vi "ArcadeJoystick.vi"(6 "Max Output":dbl=1.0, 7 "Square Inputs":bool=TRUE, 9 "Y axis value":dbl, 10 "X axis value":dbl) -> (1 "Right Motor Value":dbl, 2 "Left Motor Value":dbl)   [LabVIEW 2019]
doc: "Uses a standard algorithm to map joystick axes into motor updates for arcade driving. This algorithm does not saturate over half of the range.\n\nThis software is licensed. Open the labview\\readme\\WPI Robotics Library Open Source License.txt file for more information."
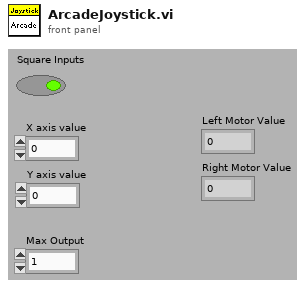
[diagram p1: front panel]
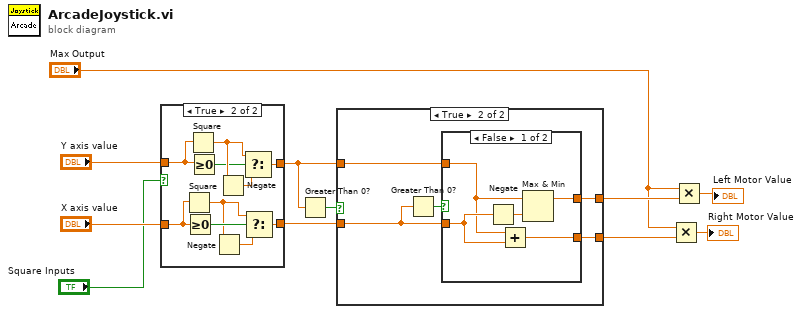
[diagram p0: block diagram]
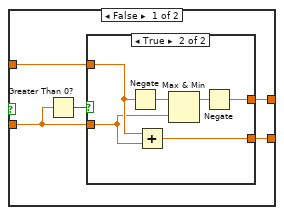
[diagram p2: hidden frame]
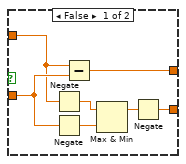
[diagram p3: hidden frame]
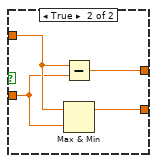
[diagram p4: hidden frame]
diagram:
  n1 = case shown="True" "Square Inputs" {
    tunnel: [w12 w23] -> w9
    tunnel: [w13 w22] -> w10
    tunnel: "X axis value" -> [w12 w21]
    tunnel: "Y axis value" -> [w13 w20]
    frame False {
    }
    frame True {
      n2 = Square(x=w21) -> (x^2=w18:dbl)
      n3 = Greater Or Equal To 0?(x=w21) -> (x >= 0?=w19:bool)
      n4 = Square(x=w20) -> (x^2=w15:dbl)
      n5 = Greater Or Equal To 0?(x=w20) -> (x >= 0?=w14:bool)
      n6 = Negate(x=w18) -> (-x=w17:dbl)
      n7 = Negate(x=w15) -> (-x=w16:dbl)
      n8 = Select(t=w15, s=w14, f=w16) -> (s? t:f=w22:dbl)
      n9 = Select(t=w18, s=w19, f=w17) -> (s? t:f=w23:dbl)
    }
  }
  n10 = Greater Than 0?(x=w10) -> (x > 0?=w11:bool)
  n11 = case shown="True" w11 {
    tunnel: w9 -> [w27 w45]
    tunnel: w10 -> [w26 w44]
    tunnel: [w25 w43] -> w8
    tunnel: [w24 w42] -> w5
    frame False {
      n12 = Greater Than 0?(x=w27) -> (x > 0?=w28:bool)
      n13 = case shown="True" w28 {
        tunnel: w27 -> [w35 w37]
        tunnel: w26 -> [w33 w38]
        tunnel: [w29 w39] -> w25
        tunnel: [w30 w36] -> w24
        frame False {
          n14 = Negate(x=w33) -> (-x=w34:dbl)
          n15 = Negate(x=w35) -> (-x=w32:dbl)
          n16 = Subtract(x=w33, y=w35) -> (x-y=w29:dbl)
          n17 = Max & Min(x=w34, y=w32) -> (max(x,y)=w31:dbl)  [unwired: 1 out]
          n18 = Negate(x=w31) -> (-x=w30:dbl)
        }
        frame True {
          n19 = Negate(x=w38) -> (-x=w41:dbl)
          n20 = Add(x=w38, y=w37) -> (x+y=w36:dbl)
          n21 = Max & Min(x=w41, y=w37) -> (max(x,y)=w40:dbl)  [unwired: 1 out]
          n22 = Negate(x=w40) -> (-x=w39:dbl)
        }
      }
    }
    frame True {
      n23 = Greater Than 0?(x=w45) -> (x > 0?=w46:bool)
      n24 = case shown="False" w46 {
        tunnel: w45 -> [w51 w53]
        tunnel: w44 -> [w48 w54]
        tunnel: [w49 w52] -> w43
        tunnel: [w47 w55] -> w42
        frame False {
          n25 = Negate(x=w51) -> (-x=w50:dbl)
          n26 = Add(x=w48, y=w51) -> (x+y=w47:dbl)
          n27 = Max & Min(x=w48, y=w50) -> (max(x,y)=w49:dbl)  [unwired: 1 out]
        }
        frame True {
          n28 = Subtract(x=w54, y=w53) -> (x-y=w52:dbl)
          n29 = Max & Min(x=w54, y=w53) -> (max(x,y)=w55:dbl)  [unwired: 1 out]
        }
      }
    }
  }
  n30 = Multiply(x="Max Output", y=w5) -> (x*y=→"Right Motor Value":dbl)
  n31 = Multiply(x="Max Output", y=w8) -> (x*y=→"Left Motor Value":dbl)
